vi "Run_5_of_5_Tests.vi"() -> ()   [LabVIEW 2019]
uses:
  <vilib>/Rock Robotics/WPI/ThirdParty/JAS_Junk/TrajLib/Trajectory_Library.lvlib
panel:
  out "String":string
  out "All Tests Finished":bool
  out "Diff Drive Train Sim":bool
  out "Elevator Sim":bool
  out "DARE - Ricatti":bool
  out "Discretization":bool
  # "FORMAL TRAJECTORY / CONTROL LIBRARY TEST PROCEDURE"
  # "Elipt Region Constraint"
  # "FUNCTION NOT\nIMPLEMENTED"
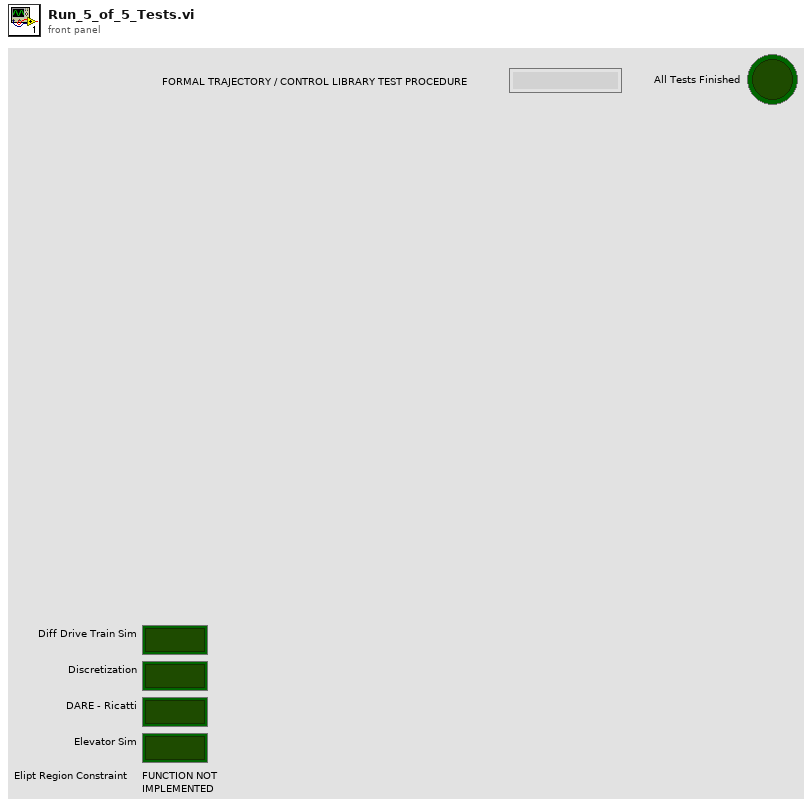
[diagram p1: front panel]
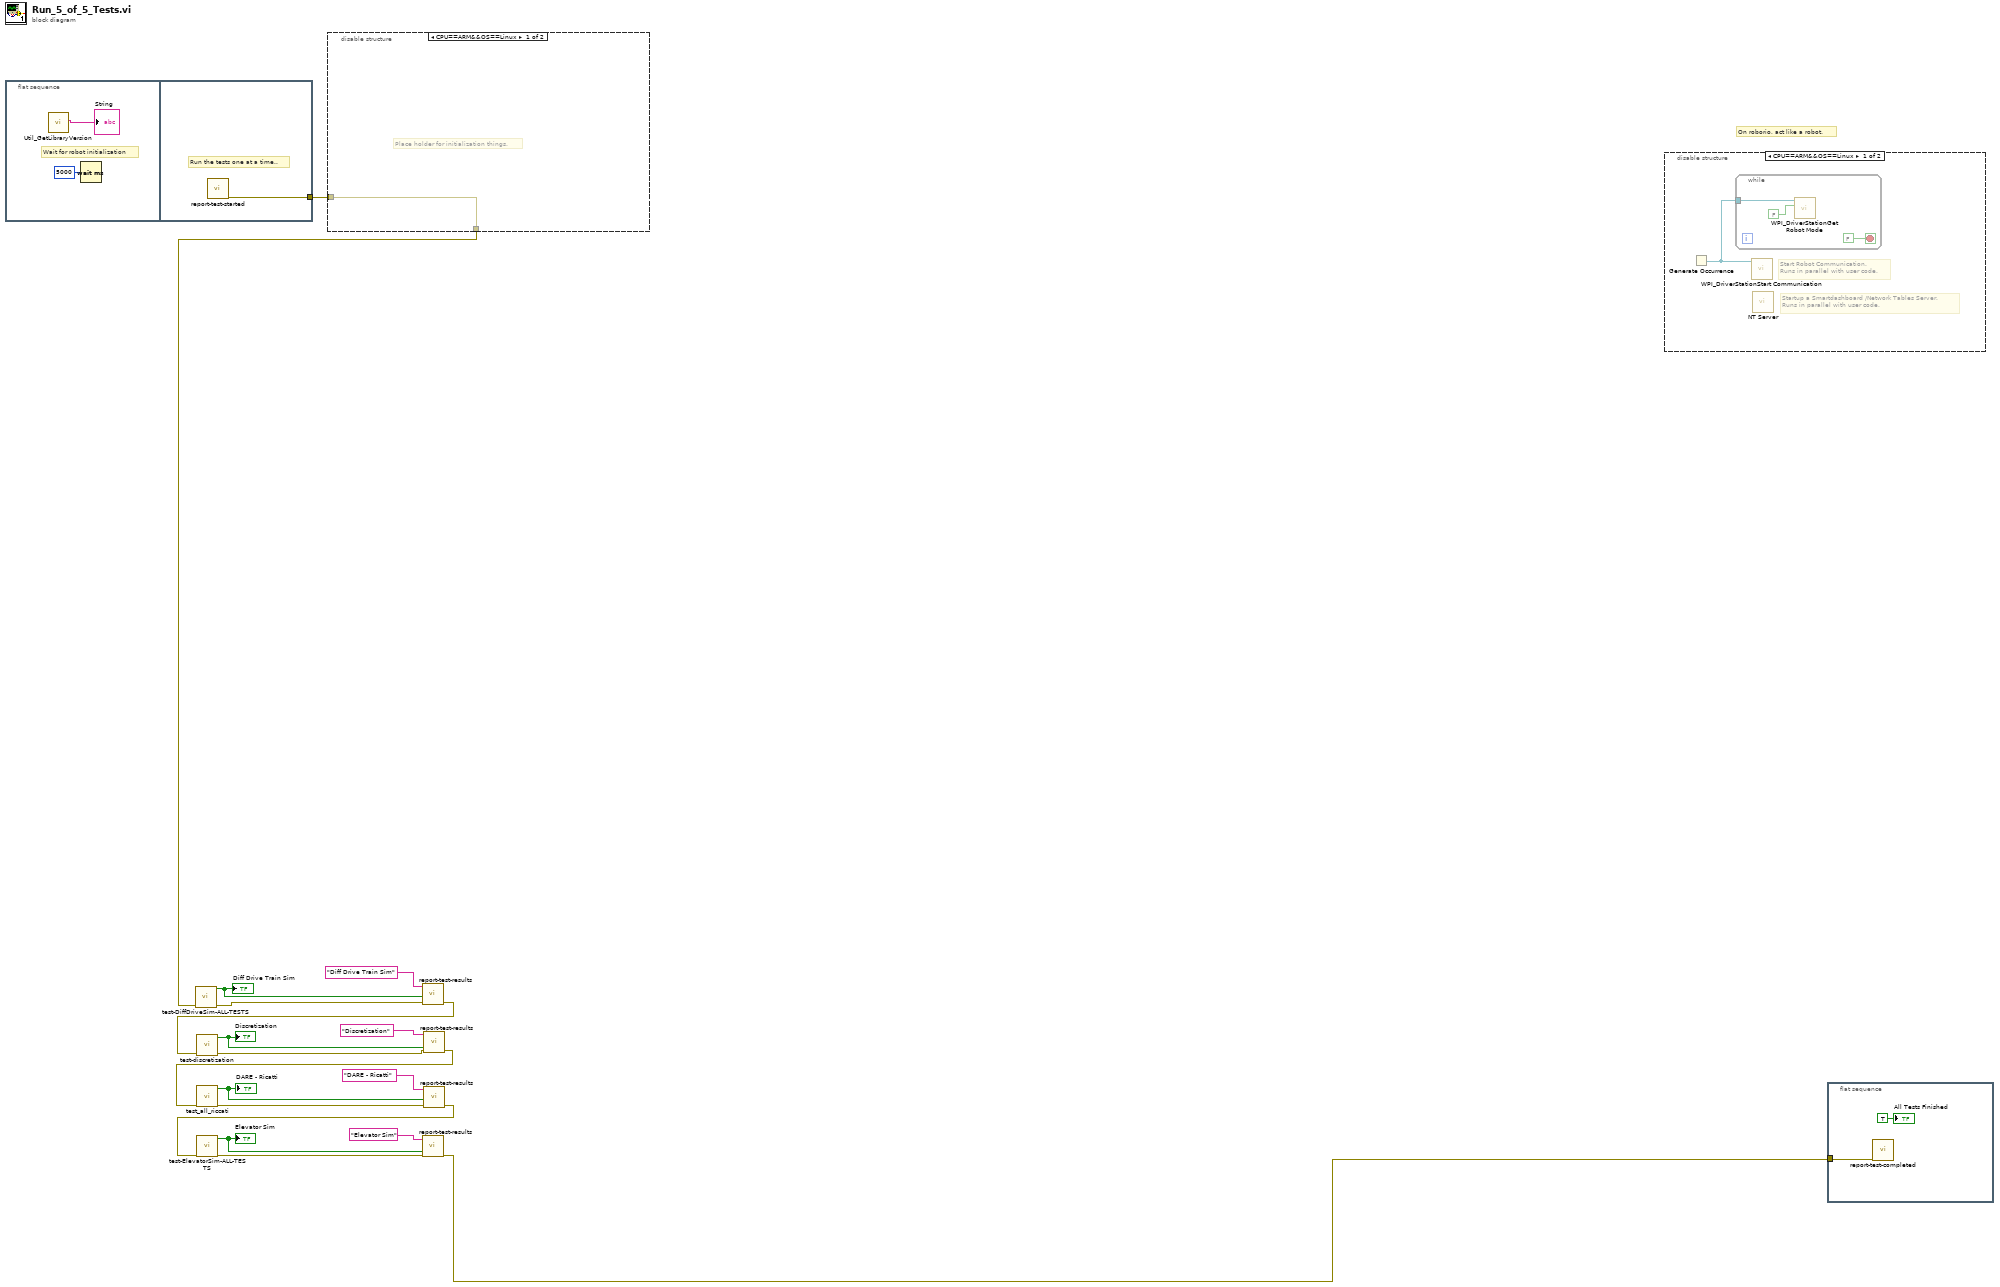
[diagram p0: block diagram]
diagram:
  # "On roborio, act like a robot."
  n1 = flat-sequence {
    tunnel: [w21] -> w3
    frame #0 {
      # "Wait for robot initialization"
      n2 = call <vilib>:"Util_GetLibraryVersion.vi"() -> ("TrajLibVersion"=→"String":string)  [unwired: 11 in]
      n3 = Wait (ms)(milliseconds to wait=u32 5000) -> ()  [unwired: 1 out]
    }
    frame #1 {
      # "Run the tests one at a time.."
      n4 = call "report-test-started.vi"() -> ("error out"=w21:errorcluster)  [unwired: 11 in]
    }
  }
  n5 = disable-structure shown="CPU==ARM&&OS==Linux" {
    disable-tunnel: w3 -> [w22 w23]
    disable-tunnel: [w22 w23] -> w1
    frame condition #0 {
      # "Place holder for initialization things."
    }
    frame condition #1 (active) {
    }
  }
  n6 = call "test-DiffDriveSim-ALL-TESTS.vi"("error in (no error)"=w1) -> ("error out"=w8:errorcluster, "All Passed"=w15:bool)  [unwired: 9 in]
  "Diff Drive Train Sim" <- w15
  n7 = call "report-test-results.vi"("error in (no error)"=w8, "TestPassed"=w15, "Test Name"="Diff Drive Train Sim") -> ("error out"=w4:errorcluster)  [unwired: 8 in]
  n8 = call "test-discretization.vi"("error in (no error)"=w4) -> ("error out"=w10:errorcluster, "All Tests Passed"=w14:bool)  [unwired: 9 in]
  "Discretization" <- w14
  n9 = call "report-test-results.vi"("error in (no error)"=w10, "TestPassed"=w14, "Test Name"="Discretization") -> ("error out"=w9:errorcluster)  [unwired: 8 in]
  n10 = call "test_all_riccati.vi"("error in (no error)"=w9) -> ("error out"=w7:errorcluster, "All Tests Passed"=w13:bool)  [unwired: 9 in]
  "DARE - Ricatti" <- w13
  n11 = call "report-test-results.vi"("error in (no error)"=w7, "TestPassed"=w13, "Test Name"="DARE - Ricatti") -> ("error out"=w5:errorcluster)  [unwired: 8 in]
  n12 = call "test-ElevatorSim-ALL-TESTS.vi"("error in (no error)"=w5) -> ("error out"=w6:errorcluster, "All Passed"=w11:bool)  [unwired: 9 in]
  "Elevator Sim" <- w11
  n13 = call "report-test-results.vi"("error in (no error)"=w6, "TestPassed"=w11, "Test Name"="Elevator Sim") -> ("error out"=w2:errorcluster)  [unwired: 8 in]
  n14 = disable-structure shown="CPU==ARM&&OS==Linux" {
    frame condition #0 {
      # "Startup a Smartdashboard /Network Tables Server.\nRuns in parallel with user code."
      # "Start Robot Communication.\nRuns in parallel with user code."
      n15 = Generate Occurrence() -> (w24:refnum<k4>)
      n16 = while {
        tunnel: w24 -> [w27]
        stop <- FALSE stop-if-true
        n17 = call <vilib>:"WPI_DriverStationGet Robot Mode.vi"("Finish"=FALSE, "DS Occurrence"=w27) -> ()  [unwired: 10 out]
      }
      n18 = call <vilib>:"WPI_DriverStationStart Communication.vi"("occurrence"=w24) -> ()  [unwired: 2 in, 9 out]
      n19 = call <vilib>:"NT Server.vi"() -> ()  [unwired: 12 in]
    }
    frame condition #1 (active) {
    }
  }
  n20 = flat-sequence {
    tunnel: w2 -> [w28]
    frame #0 {
      n21 = call "report-test-completed.vi"("error in (no error)"=w28) -> ()  [unwired: 10 in, 1 out]
      "All Tests Finished" <- TRUE ("All Tests Finished")
    }
  }
